vi "HelloWorld.vi"() -> ()   [LabVIEW 2018]
panel:
  in  "Name":string="World"
  out "response":string
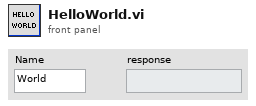
[diagram p1: front panel]
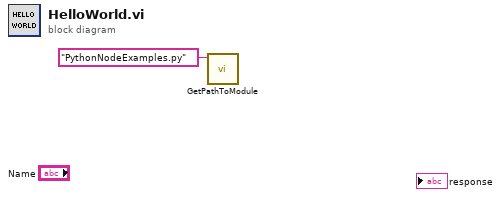
[diagram p0: block diagram]
diagram:
  n1 = call "GetPathToModule.vi"("module name"="PythonNodeExamples.py") -> ()  [unwired: 10 in, 1 out]
